vi "IndexType.vi"(0 "Axis In":T2, 5 "Index (0)":T1, 7 "Index Type":T3 items=["Incremental", "Absolute", "Registration", "Jog"], 11 "error in (no error)":errorcluster) -> (4 "Axis Out":T2, 6 "Index (duplicate)":T1, 15 "error out":errorcluster)   [LabVIEW 2009]
uses:
  typedefs/AxisSelect_Enum.ctl
  typedefs/Ultra3000/Index_Numeric.ctl
  typedefs/Ultra3000/IndexType.ctl
  typedefs/Ultra3000/Cmds.ctl
  typedefs/Ultra3000/Func.ctl
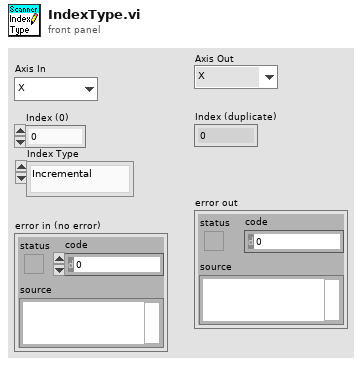
[diagram p1: front panel]
types:
  T1 = typedef "Index_Numeric.ctl" = u8
  T2 = typedef "AxisSelect_Enum.ctl" = enum16{"X", "Y", "Z", "Axis Space"}
  T3 = typedef "IndexType.ctl" = i32
  T4 = typedef "Func.ctl" = u16
  T5 = typedef "Cmds.ctl" = u16
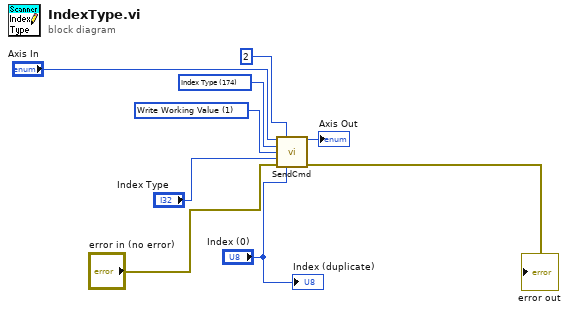
[diagram p0: block diagram]
diagram:
  w8 = T4 1 items=["Read Working Value", "Write Working Value", "Read Non-Volatile Value", "Write Non-Volatile and Woring Value", "Copy Non-Volatile Value to Working Value", "Copy Working Value to Non-Volatile Value", "Read Default Value", "Copy Default Value to Non-Volatile and Working Values", "Read Min Value", "Read Max Value", "Read Array Index Min", "Read Array Index Max"] ("Function")
  w9 = T5 174 items=["Position Command"=128, "Run Status"=117, "Fault Status"=116, "Position Error"=129, "Auto-Start Homing"=196, "Start Homing"=205, "Homing Type"=197, "Motor Position"=126, "Velocity Motor"=133, "Power-Up Status"=1, "Drive Name"=6, "Position Window Size"=22, "Position Window Time"=23, "Zero Speed Limit"=34, "Speed Window Size"=35, "Up to Speed Limit"=37, "Forward Current Limit"=47, "Reverse Current Limit"=48, "Override Mode"=67, "Operation Mode"=90, "Host Control Mode"=97, "Reset Drive"=106, "Drive Enable"=107, "Setpoint Current"=108, "Setpoint Velocity"=109, "Setpoint Acceleration"=110, "Reset Faults"=111, "Position Comparator"=349, "Postition Comparator Polarity"=350, "Position Rollover Enable"=404, "Baud Rate"=80, "Frame Format"=81, "Drive Address"=82, "Broadcast Address"=83, "Auto-start Indexing"=88, "Start Index"=112, "Host Index"=184, "Index Type"=174, "Index Dist/Pos"=175, "Index Reg Dist"=176, "Index Velocity"=177, "Index Acceleration"=178, "Index Deceleration"=179, "Index Dwell"=180, "Index Count"=181, "Index Termination"=182, "Index Pointer"=183, "Index Abort Deceleration"=185, "Positive Soft Pos Limit"=216, "Define Home"=113, "Negative Soft Pos Limit"=217] ("Command")
  n1 = call "SendCmd.vi"("Axis In"="Axis In", "Data Length Constant (0)"=u8 2, "Command"=w9, "Function"=w8, "Data (0)"="Index Type", "error in (no error)"="error in (no error)", "Index (0)"="Index (0)") -> ("Axis Out"=→"Axis Out":T2, "error out"=→"error out":errorcluster)  [unwired: 5 in, 2 out]
  "Index (duplicate)" <- "Index (0)"
